vi "MQTT_Read_Published_Message.vi"(8 "error in (no error)":errorcluster, 11 "connection ID":refnum<k5>) -> (0 "error out":errorcluster, 1 "Message":string, 2 "Topic":string, 3 "connection ID out":refnum<k5>)   [LabVIEW 2025, in "DAQIO MQTT.lvlib"]
doc: "This VI reads the last published message at the selected topic. It sends acknowledge information if required by the QoS level.\n\n© 2015 - daq.io, LLC - Peter Adelhardt"
uses:
  DAQIO MQTT.lvlib
  Controls/MessageType.ctl
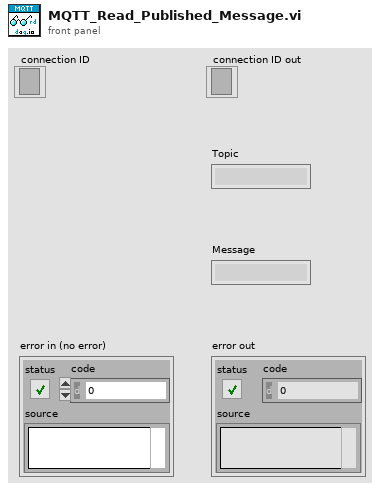
[diagram p1: front panel]
types:
  T1 = typedef "DAQIO MQTT.lvlib/MessageType.ctl" = enum32{"Reserved", "CONNECT", "CONNACK", "PUBLISH", "PUBACK", "PUBREC", "PUBREL", "PUBCOMP", "SUBSCRIBE", "SUBACK", "UNSUBSCRIBE", "UNSUBACK", "PINGREQ", "PINGRESP", "DISCONNECT", "Reserved2"}
  T2 = enum8{"At most once", "At least once", "Exactly once", "Reserved"}
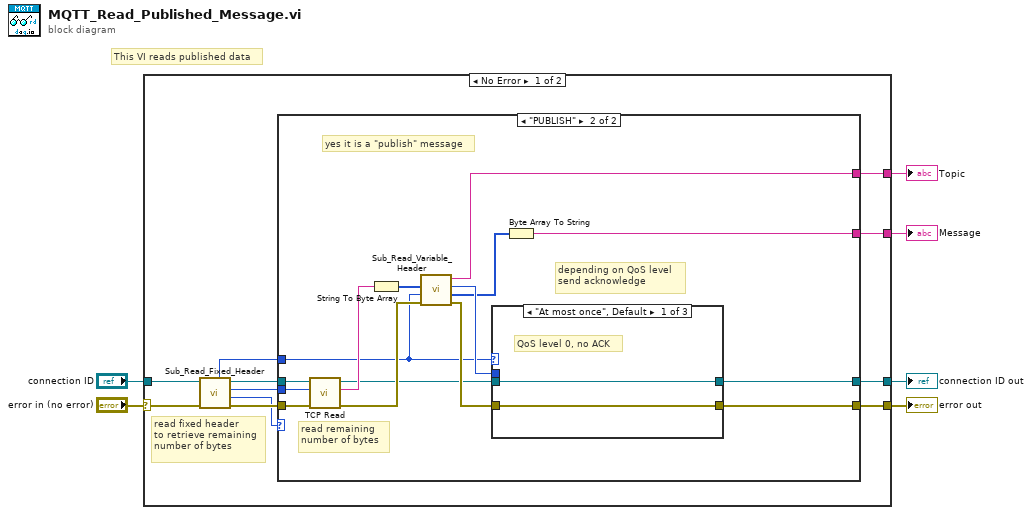
[diagram p0: block diagram]
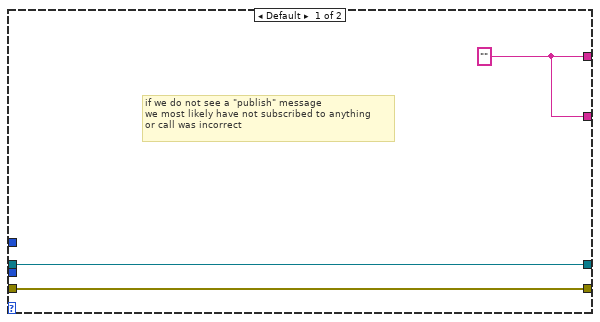
[diagram p2: hidden frame]
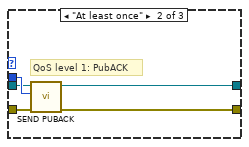
[diagram p3: hidden frame]
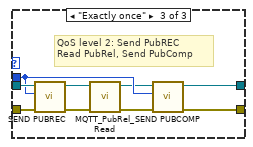
[diagram p4: hidden frame]
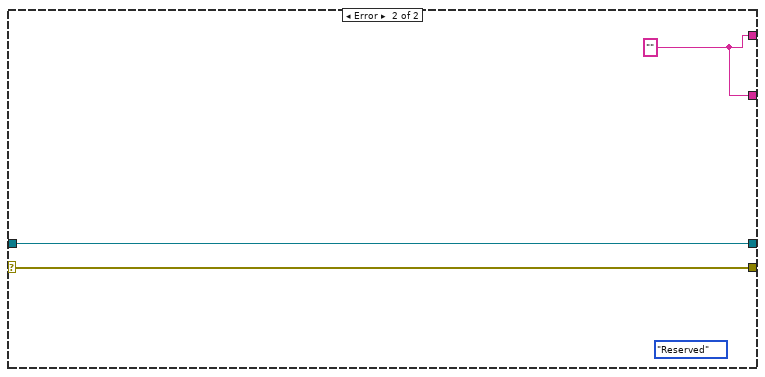
[diagram p5: hidden frame]
diagram:
  # "This VI reads published data"
  n1 = case shown="No Error" "error in (no error)" {
    selector: "error in (no error)" -> [w17 w54]
    tunnel: [w12 w54] -> w5
    tunnel: "connection ID" -> [w11 w53]
    tunnel: [w10 w53] -> w3
    tunnel: [w9 w52] -> w1
    tunnel: [w8 w52] -> w2
    frame No Error {
      # "read fixed header \nto retrieve remaining\nnumber of bytes"
      n2 = call "Sub_Read_Fixed_Header.vi"("error in (no error)"=w17, "connection ID"=w11) -> ("error out"=w14:errorcluster, "MessageType"=w7:T1, "Remaining Length"=w16:u32, "connection ID out"=w15:refnum<k5>, "QoS Level"=w13:T2)  [unwired: 3 in, 2 out]
      n3 = case shown="\"PUBLISH\"" w7 {
        tunnel: w16 -> [_ w33]
        tunnel: w15 -> [w20 w32]
        tunnel: w14 -> [w19 w31]
        tunnel: w13 -> [_ w27]
        tunnel: [w20 w25] -> w10
        tunnel: [w19 w24] -> w12
        tunnel: [w18 w23] -> w9
        tunnel: [w18 w21] -> w8
        frame Default {
          w18 = "" ("Topic Name")
          # "if we do not see a \"publish\" message\nwe most likely have not subscribed to anything\nor call was incorrect"
        }
        frame "PUBLISH" {
          # "yes it is a \"publish\" message"
          # "depending on QoS level\nsend acknowledge"
          # "read remaining\nnumber of bytes"
          n4 = call "TCP Read.vi"("error in (no error)"=w31, "bytes to read"=w33, "connection ID"=w32) -> ("error out"=w28:errorcluster, "data out"=w30:string, "connection ID out"=w26:refnum<k5>)  [unwired: 6 in]
          n5 = String To Byte Array(string=w30) -> (unsigned byte array=w29:u8[])
          n6 = call "Sub_Read_Variable_Header.vi"("error in (no error)"=w28, "QoS"=w27, "Variable Header"=w29) -> ("error out"=w34:errorcluster, "remaining bytes"=w22:u8[], "Message ID"=w35:u16, "Topic Name"=w23:string)  [unwired: 5 in]
          n7 = case shown="\"At most once\", Default" w27 {
            tunnel: w35 -> [_ w42 w47]
            tunnel: w34 -> [w36 w41 w51]
            tunnel: w26 -> [w37 w40 w50]
            tunnel: [w37 w39 w49] -> w25
            tunnel: [w36 w38 w48] -> w24
            frame "At most once", Default {
              # "QoS level 0, no ACK"
            }
            frame "At least once" {
              # "QoS level 1: PubACK"
              n8 = call "SEND PUBACK.vi"("error in (no error)"=w41, "Message ID"=w42, "connection ID"=w40) -> ("error out"=w38:errorcluster, "connection ID out"=w39:refnum<k5>)  [unwired: 6 in, 1 out]
            }
            frame "Exactly once" {
              # "QoS level 2: Send PubREC\nRead PubRel, Send PubComp"
              n9 = call "SEND PUBREC.vi"("error in (no error)"=w51, "Message ID"=w47, "connection ID"=w50) -> ("error out"=w44:errorcluster, "connection ID out"=w43:refnum<k5>)  [unwired: 7 in]
              n10 = call "MQTT_PubRel_Read.vi"("error in (no error)"=w44, "connection ID"=w43) -> ("error out"=w45:errorcluster, "connection ID out"=w46:refnum<k5>)  [unwired: 7 in, 1 out]
              n11 = call "SEND PUBCOMP.vi"("error in (no error)"=w45, "Message ID"=w47, "connection ID"=w46) -> ("error out"=w48:errorcluster, "connection ID out"=w49:refnum<k5>)  [unwired: 7 in]
            }
          }
          n12 = Byte Array To String(unsigned byte array=w22) -> (string=w21:string)
        }
      }
    }
    frame Error {
      w52 = "" ("Topic Name")
      (unwired) MessageType."Reserved" ("MessageType")
    }
  }
  "error out" <- w5
  "connection ID out" <- w3
  "Message" <- w2
  "Topic" <- w1
